vi "Temperature Graph SCPI.vi"() -> ()   [LabVIEW 2011]
uses:
  Labview/Kelvinox drivers/ITCAPPS.LLB/ITCSetupArray.ctl
  Labview/Kelvinox drivers/ITCAPPS.LLB/ITCSetup.ctl
  Labview/Kelvinox drivers/ITCSUBS.LLB/ITCIO.ctl
  Labview/Kelvinox drivers/BUSGEN.LLB/OxfordAddress.ctl
  Labview/Kelvinox drivers/ITCSUBS.LLB/ITCVersion.ctl
  Global 2.vi
panel:
  out "Pressure graph":T1(graph)
  out "T4 PT2 [K]":dbl=5.3598
  out "T4 array":dbl[](array[numeric])=[5.327, 5.3231, 5.3354, 5.3194, 5.3179, 5.3336, 5.3292, 5.3212, 5.3212, 5.3156, 5.3154, 5.3266, 5.3148, 5.3177, 5.3253, 5.3492, 5.3598]
  in  "ITC Setup(write)":T2=[{"Description"="", "IO Info"={"Address"={"Com Port"=1, "ISOBUS Address"=1, "GPIB Address"=0, "Communication"=enum."ISOBUS"}, "Version"=enum."ITC503", "Ch 1 dec places"=0, "Ch 2 dec places"=0, "Ch 3 dec places"=0, "Ch1 Name"="", "Ch2 Name"="", "Ch3 Name"=""}}]
  out "Pressure [mb]":dbl=9.5802
  out "P array":dbl[](array[numeric])=[9.5836, 9.5847, 9.5841, 9.5814, 9.5805, 9.5863, 9.5793, 9.5837, 9.5825, 9.5865, 9.5807, 9.5817, 9.5803, 9.587, 9.5834, 9.5828, 9.5802]
  in  "Comments":string
  in  "stop":bool
  in  "Delay (min.)":dbl=0.1
  in  "Record":bool
  in  "File Name":path
  out "Temperature graph":T1(graph)
  out "Rate T1 [K/Hour]":dbl=-0.21846724039143606 format="%#_4g"
  out "T1 Sample [K]":dbl=4.7873
  out "T2 VTI [K]":dbl=4.8035
  out "T3 Magnet [K]":dbl=5.3479
  out "Time":string="09:29:10"
  out "Time":dbl[](array[numeric])=[3580442914.432409, 3580442915.7414837, 3580442916.974554, 3580442918.2436266, 3580442919.4956985, 3580442920.769771, 3580442921.987841, 3580442923.209911, 3580442924.470983, 3580442925.7220545, 3580442926.9741263, 3580442928.243199, 3580442929.4662685, 3580442930.7693434, 3580442937.4147234, 3580442944.021101, 3580442950.6124783]
  out "T2 array":dbl[](array[numeric])=[4.8069, 4.8068, 4.8066, 4.8064, 4.8063, 4.806, 4.806, 4.8058, 4.8056, 4.8056, 4.8055, 4.8053, 4.8051, 4.8049, 4.8041, 4.8036, 4.8035]
  out "T1 array":dbl[](array[numeric])=[4.7915, 4.7913, 4.7911, 4.7909, 4.7907, 4.7905, 4.7903, 4.7902, 4.79, 4.7899, 4.7897, 4.7896, 4.7894, 4.7892, 4.7884, 4.7877, 4.7873]
  out "REC memory":bool
  out "T3 array":dbl[](array[numeric])=[5.3454, 5.3418, 5.3458, 5.343, 5.3399, 5.343, 5.3384, 5.3393, 5.3412, 5.3382, 5.3422, 5.3414, 5.3399, 5.3427, 5.34, 5.3432, 5.3479]
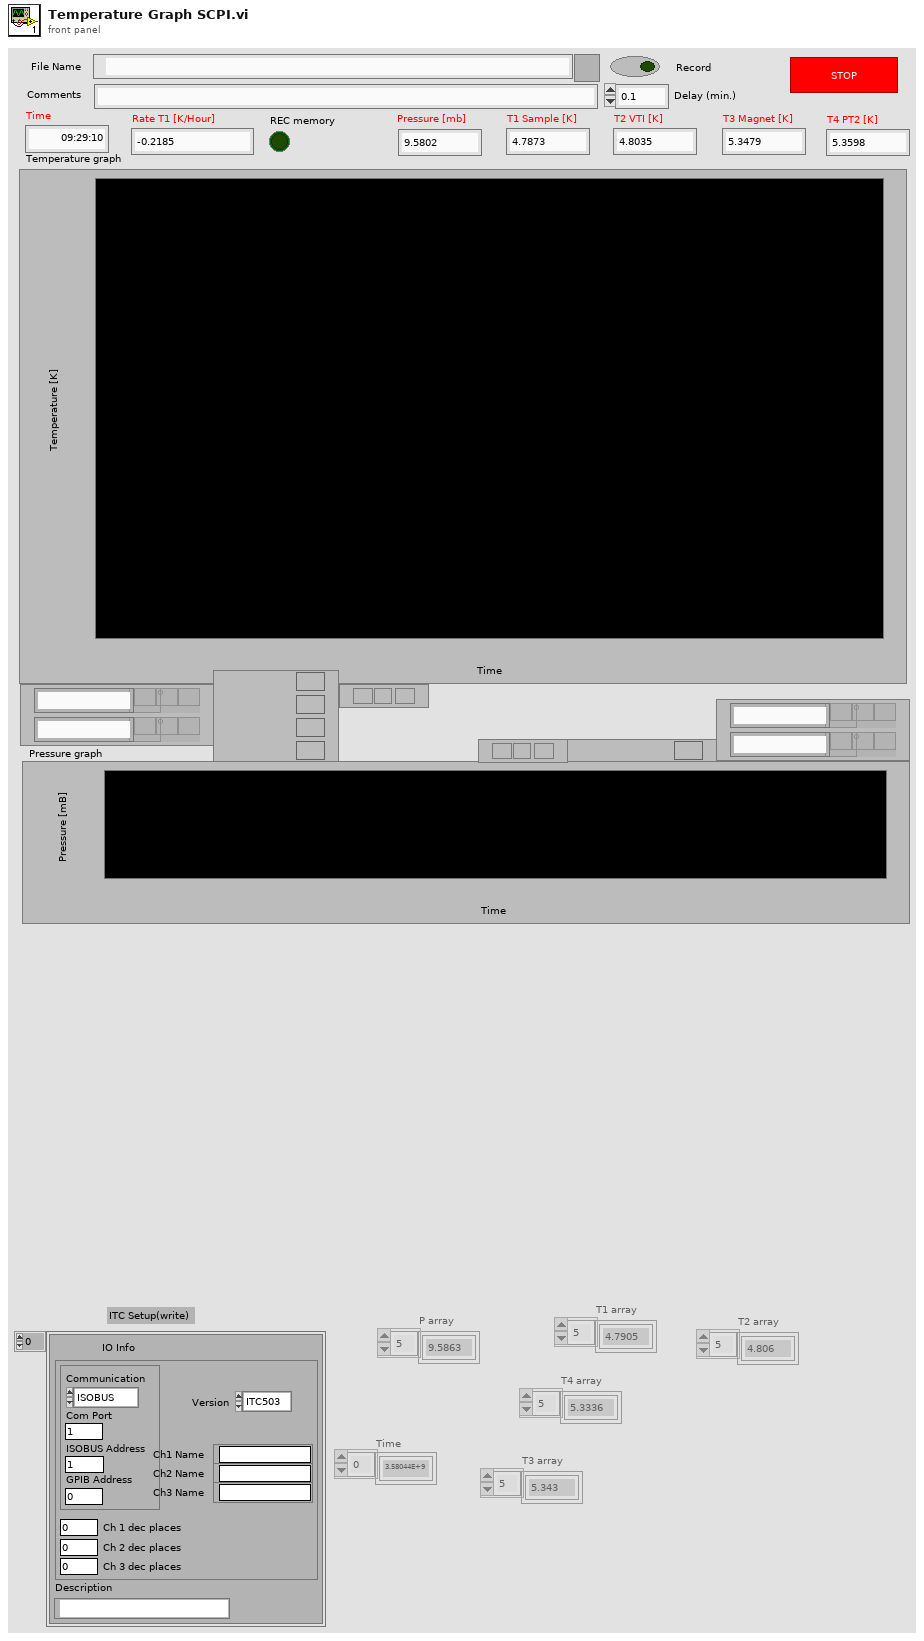
[diagram p1: front panel]
types:
  T1 = cluster{"Control X axis":dbl[], "Control Y axis":dbl[]}[]
  T2 = typedef "ITCSetupArray.ctl" = T3[]
  T3 = typedef "ITCSetup.ctl" = cluster{"Description":string, "IO Info":T4}
  T4 = typedef "ITCIO.ctl" = cluster{"Address":T5, "Version":T6, "Ch 1 dec places":i16, "Ch 2 dec places":i16, "Ch 3 dec places":i16, "Ch1 Name":string, "Ch2 Name":string, "Ch3 Name":string}
  T5 = typedef "OxfordAddress.ctl" = cluster{"Com Port":i32, "ISOBUS Address":i32, "GPIB Address":i16, "Communication":enum16{"RS232", "ISOBUS", "GPIB", "Gateway"}}
  T6 = typedef "ITCVersion.ctl" = enum16{"ITC502", "ITC503", "ITC601"}
  T7 = cluster{"ITC Setup(write)[0]":T3, "ITC Setup(write)[1]":T3, "ITC Setup(write)[2]":T3, "ITC Setup(write)[3]":T3, "ITC Setup(write)[4]":T3, "ITC Setup(write)[5]":T3, "ITC Setup(write)[6]":T3, "ITC Setup(write)[7]":T3, "ITC Setup(write)[8]":T3}
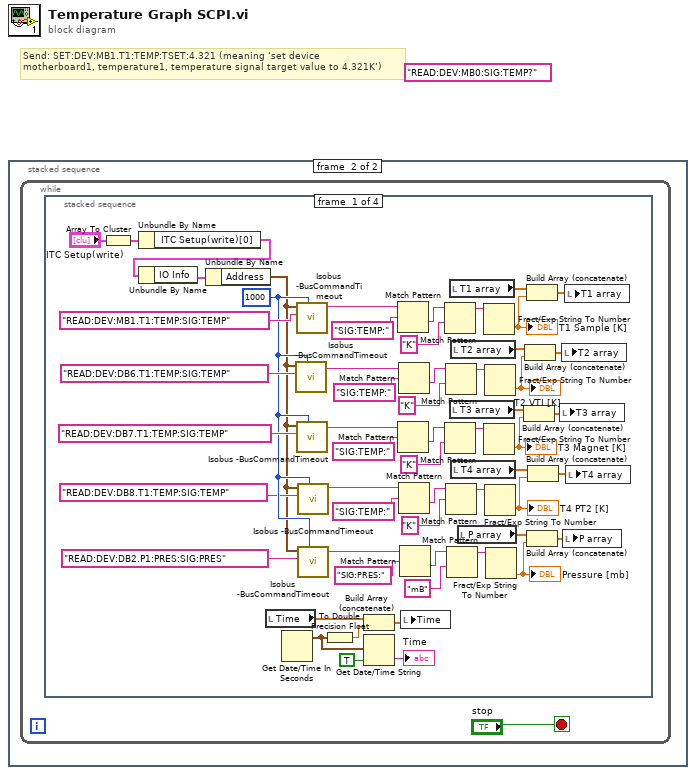
[diagram p0: block diagram]
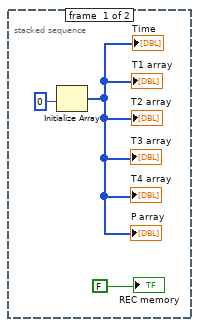
[diagram p2: hidden frame]
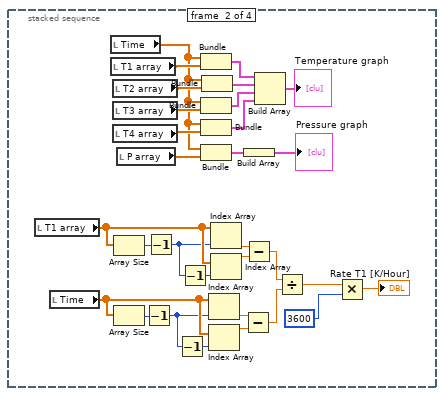
[diagram p3: hidden frame]
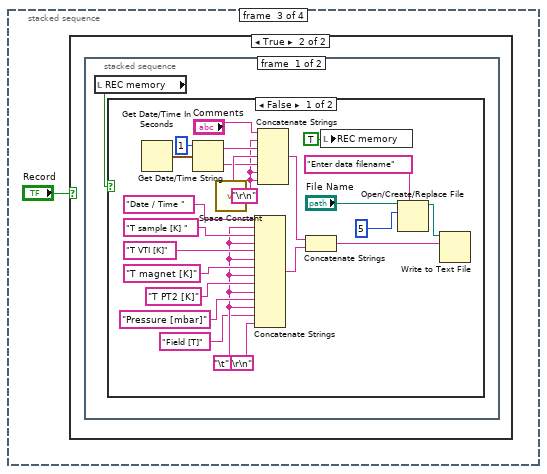
[diagram p4: hidden frame]
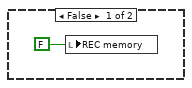
[diagram p5: hidden frame]
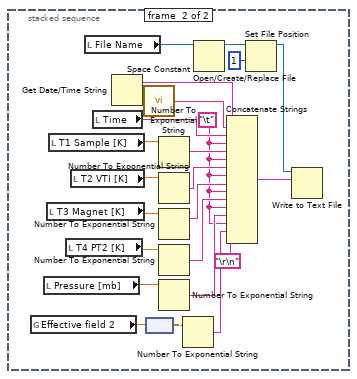
[diagram p7: hidden frame]
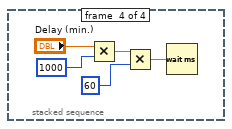
[diagram p8: hidden frame]
diagram:
  (unwired) "READ:DEV:MB0:SIG:TEMP?"
  # "Send: SET:DEV:MB1.T1:TEMP:TSET:4.321 (meaning ‘set device\nmotherboard1, temperature1, temperature signal target value to 4.321K’)"
  n1 = stacked-sequence {
    frame #0 {
      n2 = Initialize Array(0) -> (→"Time" →"T2 array" →"T1 array" →"T3 array" →"P array" →"T4 array":i32[])  [unwired: 1 in]
      "REC memory" <- FALSE
    }
    frame #1 {
      n3 = while {
        stop <- "stop" stop-if-true
        n4 = stacked-sequence {
          frame #0 {
            w8 = u32 1000
            n5 = Array To Cluster(array="ITC Setup(write)") -> (cluster=w46:T7)
            n6 = Unbundle By Name(w46) -> ("ITC Setup(write)[0]"=w44:T3)
            n7 = Unbundle By Name(w44) -> ("IO Info"=w45:T4)
            n8 = Unbundle By Name(w45) -> ("Address"=w5:T5)
            n9 = local read "Time"() -> (w61:dbl[])
            n10 = Get Date/Time In Seconds() -> (seconds since 1Jan1904=w58:timestamp)
            n11 = call "Isobus -BusCommandTimeout.vi"("Timeout (ms)"=w8, "Command"="READ:DEV:DB6.T1:TEMP:SIG:TEMP", "Address"=w5) -> ("Reply"=w19:string)  [unwired: 5 out]
            n12 = call "Isobus -BusCommandTimeout.vi"("Timeout (ms)"=w8, "Command"="READ:DEV:MB1.T1:TEMP:SIG:TEMP", "Address"=w5) -> ("Reply"=w34:string)  [unwired: 5 out]
            n13 = call "Isobus -BusCommandTimeout.vi"("Timeout (ms)"=w8, "Command"="READ:DEV:DB7.T1:TEMP:SIG:TEMP", "Address"=w5) -> ("Reply"=w20:string)  [unwired: 5 out]
            n14 = call "Isobus -BusCommandTimeout.vi"("Timeout (ms)"=w8, "Command"="READ:DEV:DB8.T1:TEMP:SIG:TEMP", "Address"=w5) -> ("Reply"=w9:string)  [unwired: 5 out]
            n15 = call "Isobus -BusCommandTimeout.vi"("Timeout (ms)"=w8, "Command"="READ:DEV:DB2.P1:PRES:SIG:PRES", "Address"=w5) -> ("Reply"=w21:string)  [unwired: 5 out]
            n16 = To Double Precision Float(number=w58) -> (double precision float=w59:dbl)
            n17 = Build Array (concatenate)(w61, w59) -> (w60:dbl[])
            n18 = Get Date/Time String(seconds (now)=w58, want seconds? (F)=TRUE) -> (time string=→"Time":string)  [unwired: 1 in, 1 out]
            n19 = Match Pattern(string=w34, regular expression="SIG:TEMP:") -> (after substring=w37:string)  [unwired: 1 in, 3 out]
            n20 = Match Pattern(string=w20, regular expression="SIG:TEMP:") -> (after substring=w27:string)  [unwired: 1 in, 3 out]
            n21 = Match Pattern(string=w19, regular expression="SIG:TEMP:") -> (after substring=w31:string)  [unwired: 1 in, 3 out]
            n22 = Match Pattern(string=w9, regular expression="SIG:TEMP:") -> (after substring=w12:string)  [unwired: 1 in, 3 out]
            n23 = Match Pattern(string=w21, regular expression="SIG:PRES:") -> (after substring=w23:string)  [unwired: 1 in, 3 out]
            n24 = local write "Time"(w60) -> ()
            n25 = Match Pattern(string=w37, regular expression="K") -> (before substring=w39:string)  [unwired: 1 in, 3 out]
            n26 = Match Pattern(string=w27, regular expression="K") -> (before substring=w29:string)  [unwired: 1 in, 3 out]
            n27 = Match Pattern(string=w31, regular expression="K") -> (before substring=w33:string)  [unwired: 1 in, 3 out]
            n28 = Match Pattern(string=w12, regular expression="K") -> (before substring=w13:string)  [unwired: 1 in, 3 out]
            n29 = Match Pattern(string=w23, regular expression="mB") -> (before substring=w25:string)  [unwired: 1 in, 3 out]
            n30 = local read "T1 array"() -> (w50:dbl[])
            n31 = local read "T3 array"() -> (w55:dbl[])
            n32 = local read "T2 array"() -> (w52:dbl[])
            n33 = local read "T4 array"() -> (w14:dbl[])
            n34 = local read "P array"() -> (w48:dbl[])
            n35 = Fract/Exp String To Number(string=w39) -> (number=w35:dbl)  [unwired: 3 in, 1 out]
            "T1 Sample [K]" <- w35
            n36 = Fract/Exp String To Number(string=w29) -> (number=w17:dbl)  [unwired: 3 in, 1 out]
            "T3 Magnet [K]" <- w17
            n37 = Fract/Exp String To Number(string=w33) -> (number=w18:dbl)  [unwired: 3 in, 1 out]
            "T2 VTI [K]" <- w18
            n38 = Fract/Exp String To Number(string=w13) -> (number=w10:dbl)  [unwired: 3 in, 1 out]
            "T4 PT2 [K]" <- w10
            n39 = Fract/Exp String To Number(string=w25) -> (number=w16:dbl)  [unwired: 3 in, 1 out]
            "Pressure [mb]" <- w16
            n40 = Build Array (concatenate)(w55, w17) -> (w54:dbl[])
            n41 = Build Array (concatenate)(w52, w18) -> (w53:dbl[])
            n42 = Build Array (concatenate)(w50, w35) -> (w51:dbl[])
            n43 = Build Array (concatenate)(w48, w16) -> (w49:dbl[])
            n44 = Build Array (concatenate)(w14, w10) -> (w15:dbl[])
            n45 = local write "T3 array"(w54) -> ()
            n46 = local write "T2 array"(w53) -> ()
            n47 = local write "P array"(w49) -> ()
            n48 = local write "T1 array"(w51) -> ()
            n49 = local write "T4 array"(w15) -> ()
          }
          frame #1 {
            n50 = local read "T1 array"() -> (w79:dbl[])
            n51 = local read "Time"() -> (w80:dbl[])
            n52 = local read "Time"() -> (w65:dbl[])
            n53 = local read "T1 array"() -> (w87:dbl[])
            n54 = local read "T2 array"() -> (w86:dbl[])
            n55 = local read "T3 array"() -> (w85:dbl[])
            n56 = local read "T4 array"() -> (w67:dbl[])
            n57 = Array Size(array=w79) -> (size(s)=w84:i32)
            n58 = Array Size(array=w80) -> (size(s)=w72:i32)
            n59 = local read "P array"() -> (w64:dbl[])
            n60 = Decrement(x=w72) -> (x-1=w71:i32)
            n61 = Decrement(x=w84) -> (x-1=w75:i32)
            n62 = Decrement(x=w71) -> (x-1=w83:i32)
            n63 = Decrement(x=w75) -> (x-1=w74:i32)
            n64 = Bundle("Time"=w65, "T1 array"=w87) -> (w91:cluster{"Time":dbl[], "T1 array":dbl[]})  [unwired: 1 in]
            n65 = Bundle("Time"=w65, "T3 array"=w85) -> (w89:cluster{"Time":dbl[], "T3 array":dbl[]})  [unwired: 1 in]
            n66 = Bundle("Time"=w65, "T4 array"=w67) -> (w66:cluster{"Time":dbl[], "T4 array":dbl[]})  [unwired: 1 in]
            n67 = Bundle("Time"=w65, "P array"=w64) -> (w63:cluster{"Time":dbl[], "P array":dbl[]})  [unwired: 1 in]
            n68 = Bundle("Time"=w65, "T2 array"=w86) -> (w90:cluster{"Time":dbl[], "T2 array":dbl[]})  [unwired: 1 in]
            n69 = Index Array(array=w80, index=w71) -> (element=w82:dbl)
            n70 = Index Array(array=w80, index=w83) -> (element=w81:dbl)
            n71 = Index Array(array=w79, index=w75) -> (element=w76:dbl)
            n72 = Index Array(array=w79, index=w74) -> (element=w73:dbl)
            n73 = Subtract(x=w82, y=w81) -> (x-y=w77:dbl)
            n74 = Build Array(w63) -> (→"Pressure graph":cluster{"Time":dbl[], "P array":dbl[]}[])
            n75 = Subtract(x=w76, y=w73) -> (x-y=w78:dbl)
            n76 = Build Array(w91, w90, w89, w66) -> (→"Temperature graph":cluster{"Time":dbl[], "T4 array":dbl[]}[])
            n77 = Divide(x=w78, y=w77) -> (x/y=w70:dbl)
            n78 = Multiply(x=w70, y=3600) -> (x*y=→"Rate T1 [K/Hour]":dbl)
          }
          frame #2 {
            n79 = case shown="True" "Record" {
              frame False {
                n80 = local write "REC memory"(FALSE) -> ()
              }
              frame True {
                n81 = stacked-sequence {
                  frame #0 {
                    n82 = local read "REC memory"() -> (w94:bool)
                    n83 = case shown="False" w94 {
                      frame False {
                        w100 = "\r\n"
                        w97 = "\t"
                        n84 = Get Date/Time In Seconds() -> (seconds since 1Jan1904=w116:timestamp)
                        n85 = Get Date/Time String(date format (0)=1, seconds (now)=w116) -> (date string=w103:string, time string=w101:string)  [unwired: 1 in]
                        n86 = call <vilib>:"Space Constant.vi"() -> ("String"=w102:string)
                        n87 = Concatenate Strings("Date / Time ", w97, "T sample [K] ", w97, "T VTI [K]" ("chaîne"), w97, "T magnet [K]" ("chaîne"), w97, "T PT2 [K]" ("chaîne"), w97, "Pressure [mbar]" ("chaîne"), w97, "Field [T]" ("chaîne"), "\r\n") -> (w113:string)
                        n88 = Concatenate Strings("Comments", w100, w103, w102, w101, w100, w100) -> (w114:string)
                        n89 = Concatenate Strings(w114, w113) -> (w112:string)
                        n90 = local write "REC memory"(TRUE) -> ()
                        n91 = Open/Create/Replace File(file path (use dialog)="File Name", prompt="Enter data filename", operation (0:open)=5) -> (refnum out=w105:refnum<file>)  [unwired: 3 in, 2 out]
                        n92 = Write to Text File(file (use dialog)=w105, text=w112) -> ()  [unwired: 2 in, 3 out]
                      }
                      frame True {
                      }
                    }
                  }
                  frame #1 {
                    w123 = "\t"
                    n93 = global read "Global 2.vi" "Effective field 2"() -> (w120:dbl[unit])
                    n94 = local read "Pressure [mb]"() -> (w121:dbl)
                    n95 = local read "T3 Magnet [K]"() -> (w135:dbl)
                    n96 = local read "T1 Sample [K]"() -> (w137:dbl)
                    n97 = local read "T4 PT2 [K]"() -> (w129:dbl)
                    n98 = local read "T2 VTI [K]"() -> (w141:dbl)
                    n99 = local read "File Name"() -> (w134:path)
                    n100 = local read "Time"() -> (w130:string)
                    n101 = Get Date/Time String() -> (date string=w126:string)  [unwired: 3 in, 1 out]
                    n102 = call <vilib>:"Space Constant.vi"() -> ("String"=w125:string)
                    n103 = node(w120) -> (w119:dbl)
                    n104 = Number To Exponential String(number=w137) -> (E-format string=w138:string)  [unwired: 3 in]
                    n105 = Number To Exponential String(number=w141) -> (E-format string=w140:string)  [unwired: 3 in]
                    n106 = Number To Exponential String(number=w135) -> (E-format string=w139:string)  [unwired: 3 in]
                    n107 = Number To Exponential String(number=w129) -> (E-format string=w127:string)  [unwired: 3 in]
                    n108 = Number To Exponential String(number=w121) -> (E-format string=w128:string)  [unwired: 3 in]
                    n109 = Number To Exponential String(number=w119) -> (E-format string=w122:string)  [unwired: 3 in]
                    n110 = Open/Create/Replace File(file path (use dialog)=w134) -> (refnum out=w133:refnum<file>)  [unwired: 5 in, 2 out]
                    n111 = Concatenate Strings(w126, w125, w130, w123, w138, w123, w140, w123, w139, w123, w127, w123, w128, w123, w122, "\r\n") -> (w136:string)
                    n112 = Set File Position(refnum=w133, from (0:start)=1) -> (refnum out=w132:refnum<file>)  [unwired: 2 in, 1 out]
                    n113 = Write to Text File(file (use dialog)=w132, text=w136) -> ()  [unwired: 2 in, 3 out]
                  }
                }
              }
            }
          }
          frame #3 {
            n114 = Multiply(x="Delay (min.)", y=1000) -> (x*y=w143:dbl)
            n115 = Multiply(x=w143, y=60) -> (x*y=w142:dbl)
            n116 = Wait (ms)(milliseconds to wait=w142) -> ()  [unwired: 1 out]
          }
        }
      }
    }
  }
